vi "Get DIDPID VS References.vi"(8 "error in (no error)":errorcluster, 10 "GUID":string, 11 "Section Ref in":T1 format="%.0x") -> (0 "error out":errorcluster, 2 "DIDPID Array":T2[](array[typedef]) {"Signal Refs" format="%.0x"}, 3 "Section Ref out":T1 format="%.0x")   [LabVIEW 2013, in "Diagnostics Addon Engine.lvlib"]
uses:
  Diagnostics Addon Engine.lvlib
  <vilib>/NI Veristand/Custom Device API/Custom Device Item Ref.ctl
  DIDPID Signal VS References.ctl
  Shared/FG Action.ctl
  <vilib>/NI Veristand/Custom Device Tools/Custom Device Utility Library/NI VeriStand - Search for Item by GUID.vi
  Shared/GUID Lookup.vi
  <vilib>/NI Veristand/Custom Device API/NI VeriStand - Get Item Property.vi
  <vilib>/NI Veristand/Custom Device API/Get Item Property (Variant).vi
  <vilib>/NI Veristand/Custom Device Tools/Custom Device Utility Library/Custom Device Utility Library.lvlib
  <vilib>/NI Veristand/Custom Device API/Custom Device API.lvlib
  Shared/Diagnostics Addon Shared.lvlib
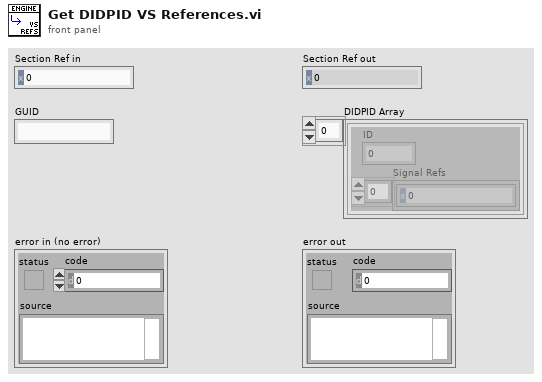
[diagram p1: front panel]
types:
  T1 = typedef "Custom Device API.lvlib/Custom Device Item Ref.ctl" = u64
  T2 = typedef "Diagnostics Addon Engine.lvlib/DIDPID Signal VS References.ctl" = cluster{"ID":u16, "Signal Refs":T1[]}
  T3 = typedef "Diagnostics Addon Shared.lvlib/FG Action.ctl" = enum16{"Get", "Set"}
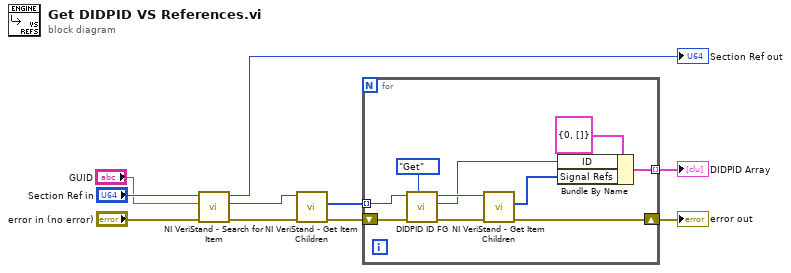
[diagram p0: block diagram]
diagram:
  n1 = call-poly <vilib>:"NI VeriStand - Search for Item.vi"("error in"="error in (no error)", "Item GUID"="GUID", "Section Ref in"="Section Ref in") -> ("error out"=w2:errorcluster, "Item Ref"=w3:T1, "Section Ref out"=→"Section Ref out":T1)  [unwired: 5 in, 1 out]
  n2 = call <vilib>:"NI VeriStand - Get Item Children.vi"("error in (no error)"=w2, "Item Ref in"=w3) -> ("error out"=w4:errorcluster, "Child Refs"=w5:T1[])  [unwired: 6 in, 2 out]
  n3 = for {
    shift-right: [w16] -> w9
    shift-left: w4 -> [w20]
    tunnel: w5 -> [w19] mode=indexing
    tunnel: [w12] -> w8 mode=indexing
    n4 = call "DIDPID ID FG.vi"("Action"=FG_Action."Get", "error in (no error)"=w20, "Device Item Ref in"=w19) -> ("error out"=w18:errorcluster, "ID"=w14:u16, "Device Item Ref out"=w17:T1)  [unwired: 6 in]
    n5 = call <vilib>:"NI VeriStand - Get Item Children.vi"("error in (no error)"=w18, "Item Ref in"=w17) -> ("error out"=w16:errorcluster, "Child Refs"=w15:T1[])  [unwired: 6 in, 2 out]
    n6 = Bundle By Name(cluster=T2 {"ID"=0, "Signal Refs"=[]}, "ID"=w14, "Signal Refs"=w15) -> (w12:T2)
  }
  "error out" <- w9
  "DIDPID Array" <- w8
